vi "cal_error_out_pos.vi"(10 "Visa Out  Position":cluster{"Left":u32, "Top":i32}, 11 "Last Function Position":cluster{"Left":i32, "Top":i32}) -> (3 "Error Out  Position":cluster{"Left":u32, "Top":i32})   [LabVIEW 2018]
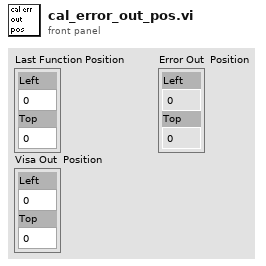
[diagram p1: front panel]
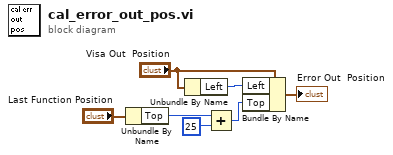
[diagram p0: block diagram]
diagram:
  n1 = Unbundle By Name("Last Function Position") -> ("Top"=w6:i32)
  n2 = Unbundle By Name("Visa Out  Position") -> ("Left"=w4:u32)
  n3 = Add(x=w6, y=25) -> (x+y=w1:i32)
  n4 = Bundle By Name(cluster="Visa Out  Position", "Left"=w4, "Top"=w1) -> (→"Error Out  Position":cluster{"Left":u32, "Top":i32})
